vi "Serialise.vi"(8 "error in (no error)":errorcluster, 11 "object in":refnum<class "Message Class.lvclass">) -> (0 "error out":errorcluster, 1 "Serialised String":string, 2 "Serialised String":string[](array[string]), 3 "object out":refnum<class "Message Class.lvclass">)   [LabVIEW 2018, in "ClientMessaging.lvlib" / "Message Class.lvclass"]
doc: "Serialise the message structure"
uses:
  Message Class.lvclass
  115712b1-f0cd-47d6-9e0b-1b149b3bba4c.vi
  3cd1b450-a124-4f29-a93f-e8aca37b2ab7.vi
  <vilib>/JDP Science/JSONtext/Variant to JSON Text.vi
  <vilib>/JDP Science/JSONtext/Set Multiple Object Items.vi
  ClientMessaging.lvlib
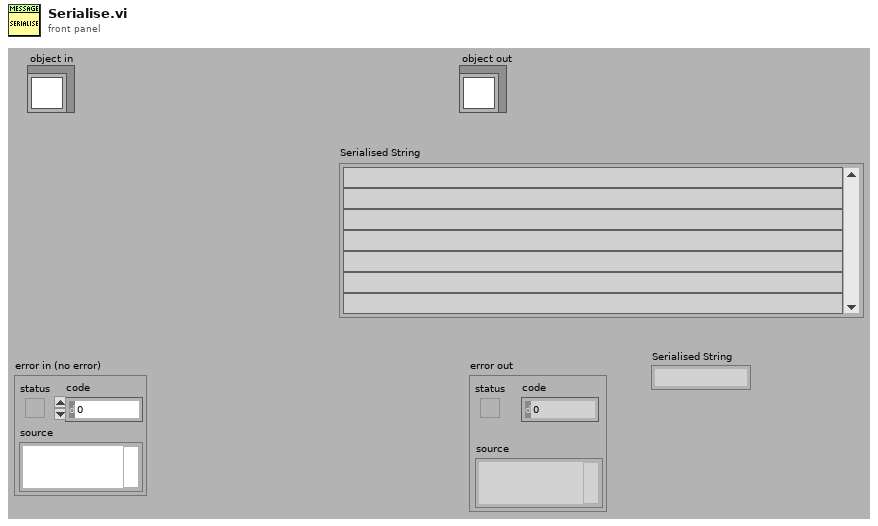
[diagram p1: front panel]
types:
  T1 = typedef "ClientMessaging.lvlib/Message Class.lvclass/header_dict.ctl" = cluster{"msg_id":string, "username":string, "session":string, "date":timestamp, "msg_type":string, "version":string}
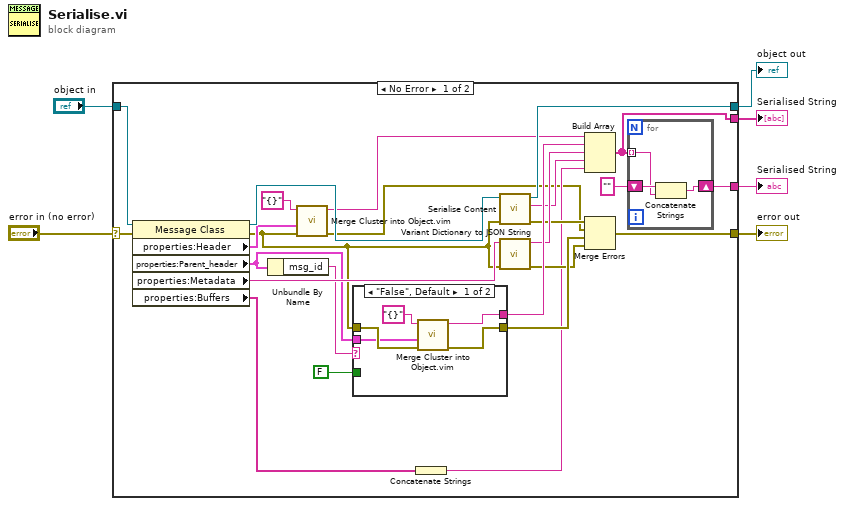
[diagram p0: block diagram]
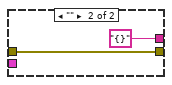
[diagram p2: hidden frame]
diagram:
  n1 = case shown="No Error" "error in (no error)" {
    selector: "error in (no error)" -> [w21 w43]
    tunnel: [w20 w43] -> w5
    tunnel: [w28 w42] -> w3
    tunnel: "object in" -> [w31 w42]
    tunnel: [w14 _] -> w2
    tunnel: [w13 _] -> w1
    frame No Error {
      n2 = property class="Message Class"(reference=w31, error in=w21) -> (reference out=w30:refnum<class "Message Class.lvclass">, error out=w9:errorcluster, "properties:Header"=w10:T1, "properties:Parent_header"=w16:T1, "properties:Metadata"=w29:string, "properties:Buffers"=w18:string[])
      n3 = Unbundle By Name(w16) -> ("msg_id"=w15:string)
      n4 = call "Merge Cluster into Object.vim"("error in (no error)"=w9, "Any Cluster"=w10, "JSON"="{}") -> ("error out"=w8:errorcluster, "<JSON>"=w7:string)  [unwired: 6 in]
      n5 = case shown="\"False\", Default" w15 {
        tunnel: w16 -> [w37 _]
        tunnel: w9 -> [w39 w40]
        tunnel: [w36 "{}" ("JSON String")] -> w27
        tunnel: [w38 w40] -> w23
        tunnel: FALSE ("Multiline (T)") -> [_ _]
        frame "False", Default {
          n6 = call "Merge Cluster into Object.vim"("error in (no error)"=w39, "Any Cluster"=w37, "JSON"="{}") -> ("error out"=w38:errorcluster, "<JSON>"=w36:string)  [unwired: 6 in]
        }
        frame "" {
        }
      }
      n7 = Concatenate Strings(w18) -> (w17:string)
      n8 = call-dynamic "Serialise Content.vi"("error in (no error)"=w9, "object in"=w30) -> ("error out"=w24:errorcluster, "Content"=w25:string, "object out"=w28:refnum<class "Message Class.lvclass">)  [unwired: 7 in]
      n9 = call "Variant Dictionary to JSON String.vi"("error in (no error)"=w9, "Registry In"=w29) -> ("error out"=w22:errorcluster, "JSON String"=w26:string)  [unwired: 8 in]
      n10 = Build Array(w7, w27, w26, w25, w17) -> (w14:string[])
      n11 = Merge Errors(w24, w8, w23, w22) -> (w20:errorcluster)
      n12 = for {
        tunnel: w14 -> [w32] mode=indexing
        shift-right: [w33] -> w13
        shift-left: "" -> [w34]
        n13 = Concatenate Strings(w34, w32) -> (w33:string)
      }
    }
    frame Error {
    }
  }
  "error out" <- w5
  "object out" <- w3
  "Serialised String" <- w2
  "Serialised String" <- w1
